vi "APOSGPS_String_To_Pos.vi"(8 "GPS IN":string="$GPGGA,080346.00,6343.152342,N,01104.396313,E,2,12,0.6,12.19,M,39.84,M,22.0,1007*4E", 11 "APOS IN":string="$PSIMSSB,170342.710,B34,A,,C,N,M,7.812,0.841,4.217,0.139,T,0.010904,") -> (2 "ROVpos":T1 caption="Real Matrix")   [LabVIEW 2012]
uses:
  <vilib>/Analysis/Matrix/Datatypes/RealMatrix.ctl
  <vilib>/imath/engines/lvmath2/RunTimeEngine/ErrorHandling/NIMS_Finalize Error.vi
  <vilib>/imath/engines/lvmath2/RunTimeEngine/Managers/WorkSpace/UID Generator.vi
  <vilib>/Analysis/Matrix/Numeric/Conversions/Matrix To Array - RM.vi
  <vilib>/imath/engines/lvmath2/RunTimeEngine/Managers/SymbolTable/Clear UID.vi
  <vilib>/imath/engines/lvmath2/RunTimeEngine/NodeEndStatement/NIMS_NodeEndStatement_Output.vi
  <instcachedir>/0/NIMS_NodeEndStatement_Output_53EC0D466D134D7ABD903AC30B43404B.lvgen/NIMS_NodeEndStatement_Output_53EC0D466D134D7ABD903AC30B43404B_012.vi
  <vilib>/Analysis/Matrix/Numeric/Conversions/Array To Matrix - RA2.vi
  <instcachedir>/0/NIMS_NodeEndStatement_Output_53EC0D466D134D7ABD903AC30B43404B.lvgen/NIMS_NodeEndStatement_Output_53EC0D466D134D7ABD903AC30B43404B_014.vi
  <vilib>/imath/engines/lvmath/Functions/Error Handling/MergeErrorsWrapper.vi
  <vilib>/imath/engines/lvmath2/RunTimeEngine/VariableToken/Read/NIMS_Get Elements - SorM(_,$) - Check.vi
  <instcachedir>/0/NIMS_Get Elements - SorM(_,$) - Check_FE352FA85B844FB785E5C28FDABD92A5.lvgen/NIMS_Get Elements - SorM(_,$) - Check_FE352FA85B844FB785E5C28FDABD92A5_000.vi
  <vilib>/imathl/engines/lvmath/Functions/Error Handling/Create Error.vi
  <vilib>/imath/engines/lvmath2/RunTimeEngine/RangeToken/NIMS_Range_R2.vi
  <vilib>/imath/engines/lvmath2/RunTimeEngine/ReplaceToken/NIMS_Replace - Check Row.vi
  <instcachedir>/0/NIMS_Replace - Check Row_8C35B66FE73A429EAC382AAA935851F0.lvgen/NIMS_Replace - Check Row_8C35B66FE73A429EAC382AAA935851F0_001.vi
  <vilib>/imath/engines/lvmath2/RunTimeEngine/ReplaceToken/NIMS_Replace - Size Check M(_,$)=VorM.vi
  <instcachedir>/0/NIMS_Replace - Size Check M(_,$)=VorM_05C8DDF28A13406EBCBD8C1ACDF4F548.lvgen/NIMS_Replace - Size Check M(_,$)=VorM_05C8DDF28A13406EBCBD8C1ACDF4F548_000.vi
  <vilib>/imath/engines/lvmath2/RunTimeEngine/ReplaceToken/NIMS_Replace - Assignment Check M(_,$)=VorM.vi
  <instcachedir>/0/NIMS_Replace - Assignment Check M(_,$)=VorM_DBF82BC42B054E2BA4F8E4D1989751AD.lvgen/NIMS_Replace - Assignment Check M(_,$)=VorM_DBF82BC42B054E2BA4F8E4D1989751AD_000.vi
  <vilib>/imath/engines/lvmath2/RunTimeEngine/VariableToken/Read/NIMS_Get Elements - RV(_) - Check.vi
  <instcachedir>/0/NIMS_Get Elements - RV(_) - Check_09E565EE58C54071A799578B82C9999A.lvgen/NIMS_Get Elements - RV(_) - Check_09E565EE58C54071A799578B82C9999A_000.vi
  <vilib>/imath/engines/lvmath2/RunTimeEngine/RunTimeType/NIMS_RunTimeType_From StrictType (excl LVString).vi
  <instcachedir>/0/NIMS_RunTimeType_From StrictType (excl LVString)_AC52D965D0864706932D20A05968E122.lvgen/NIMS_RunTimeType_From StrictType (excl LVString)_AC52D965D0864706932D20A05968E122_000.vi
  <vilib>/imath/engines/lvmath2/RunTimeEngine/ErrorHandling/NIMS_Create Error From Enums.vi
  <vilib>/imath/engines/lvmath2/RunTimeEngine/LocalVariableDefStatement/MC_LocalVariableDefStatement_Display.vi
  <vilib>/imath/engines/lvmath2/RunTimeEngine/RunTimeType/NIMS_RunTimeType_Set Source Original Bool.vi
  <vilib>/Analysis/Matrix/NI_Matrix.lvlib
  <vilib>/imath/engines/lvmath2/RunTimeEngine/Managers/SymbolTable/NIMS_WorkSpace.lvlib
panel:
  out "APOS String out":string
  out "GPS String out":string
  out "update":bool
  out "number of rows 2":i32
  out "number of rows":i32
  out "array 2":string[](array[string])
  out "array":string[](array[string])
  out "y":dbl
  out "x":dbl
  out "utmzone":string[](array[string])
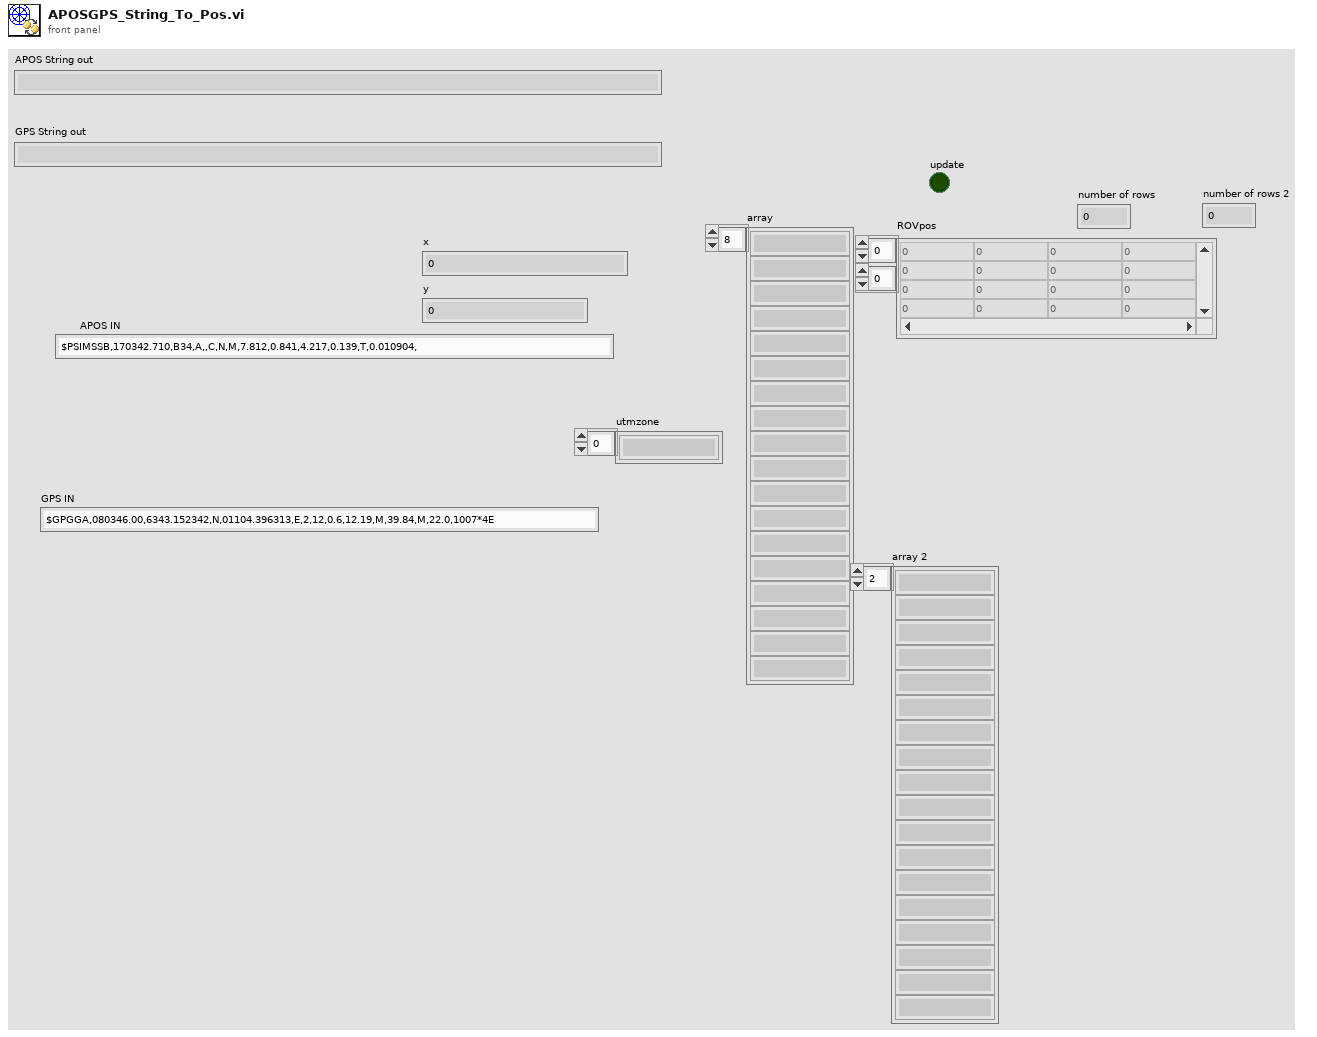
[diagram p1: front panel]
types:
  T1 = typedef "NI_Matrix.lvlib/RealMatrix.ctl" = dbl[][]
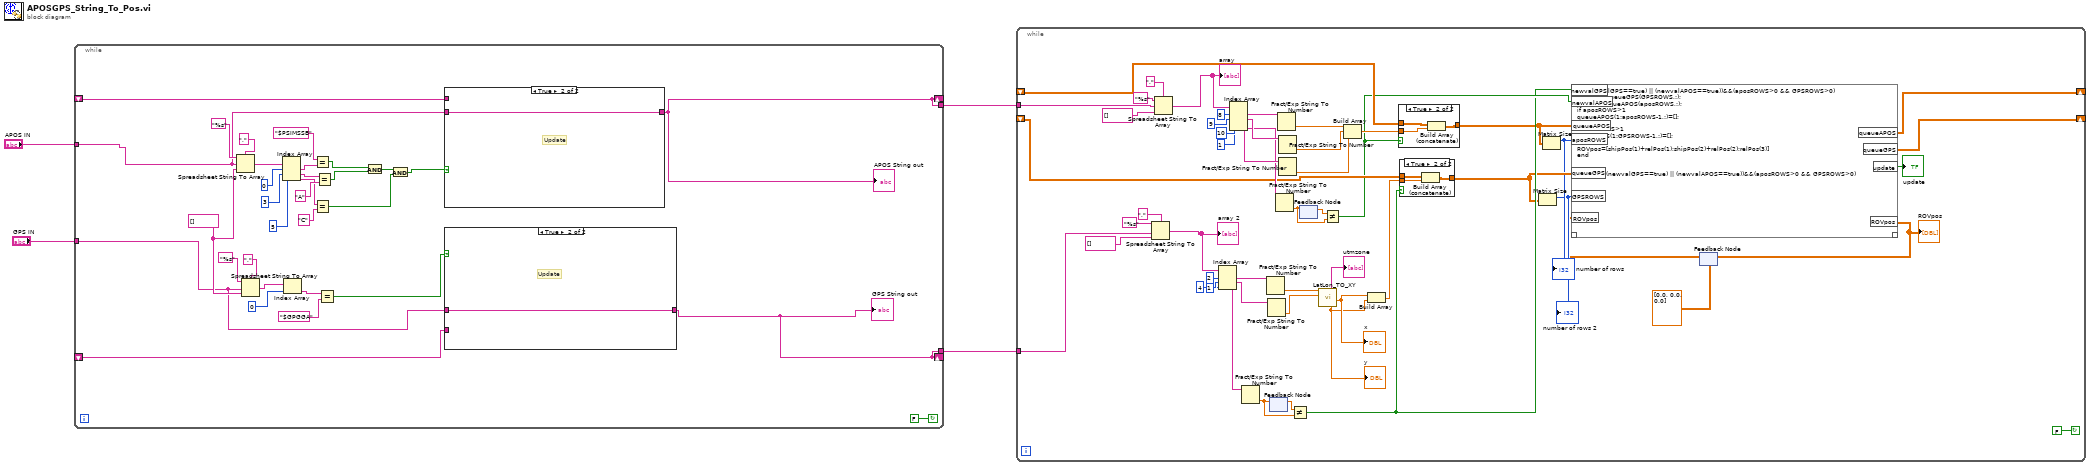
[diagram p0: block diagram]
diagram:
  n1 = while {
    shift-right: [w7] -> _
    shift-left: _ -> [w20]
    shift-right: [w8] -> _
    shift-left: _ -> [w16]
    tunnel: [w8] -> w4
    tunnel: [w7] -> w3
    tunnel: "APOS IN" -> [w6]
    tunnel: "GPS IN" -> [w5]
    stop <- FALSE continue-if-true
    w33 = string[] []
    n2 = Spreadsheet String To Array(delimiter (Tab)=",", format string="%s", spreadsheet string=w6, array type (2D Dbl)=w33) -> (array=w31:string[])
    n3 = Spreadsheet String To Array(delimiter (Tab)=",", format string="%s", spreadsheet string=w5, array type (2D Dbl)=w33) -> (array=w34:string[])
    n4 = Index Array(array=w31, index #1=0, index #2=3, index #3=5) -> (element #1=w25:string, element #2=w23:string, element #3=w13:string)
    n5 = Index Array(array=w34, index=0) -> (element=w19:string)
    n6 = Equal?(x="$PSIMSSB", y=w25) -> (x = y?=w22:bool)
    n7 = Equal?(x=w13, y="C") -> (x = y?=w10:bool)
    n8 = Equal?(x=w23, y="A") -> (x = y?=w21:bool)
    n9 = Equal?(x=w19, y="$GPGGA") -> (x = y?=w17:bool)
    n10 = And(x=w22, y=w21) -> (x .and. y?=w11:bool)
    n11 = And(x=w11, y=w10) -> (x .and. y?=w9:bool)
    n12 = case shown="True" w9 {
      tunnel: w6 -> [_ w40]
      tunnel: [w39 w40] -> w7
      tunnel: w20 -> [w39 _]
      frame False {
        # "Keep old value"
      }
      frame True {
        # "Update"
      }
    }
    "APOS String out" <- w7
    n13 = case shown="True" w17 {
      tunnel: w5 -> [_ w38]
      tunnel: [w37 w38] -> w8
      tunnel: w16 -> [w37 _]
      frame False {
        # "keep old value"
      }
      frame True {
        # "Update"
      }
    }
    "GPS String out" <- w8
  }
  n14 = while {
    shift-right: [w47] -> _
    shift-left: _ -> [w56]
    shift-right: [w46] -> _
    shift-left: _ -> [w58]
    tunnel: w4 -> [w43]
    tunnel: w3 -> [w42]
    stop <- FALSE continue-if-true
    n15 = Spreadsheet String To Array(delimiter (Tab)=",", format string="%s", spreadsheet string=w43, array type (2D Dbl)=string[] [] ("Array")) -> (array=w78:string[])
    "array 2" <- w78
    n16 = Spreadsheet String To Array(delimiter (Tab)=",", format string="%s", spreadsheet string=w42, array type (2D Dbl)=string[] [] ("Array")) -> (array=w89:string[])
    "array" <- w89
    n17 = Index Array(array=w78, index #1=2 ("index"), index #2=4 ("index"), index #3=1 ("index")) -> (element #1=w81:string, element #2=w82:string, element #3=w65:string)
    n18 = Index Array(array=w89, index #1=8 ("index"), index #2=9 ("index"), index #3=10 ("index"), index #4=1 ("index")) -> (element #1=w85:string, element #2=w84:string, element #3=w83:string, element #4=w64:string)
    n19 = Fract/Exp String To Number(string=w65) -> (number=w60:dbl)  [unwired: 3 in, 1 out]
    n20 = Fract/Exp String To Number(string=w81) -> (number=w74:dbl)  [unwired: 3 in, 1 out]
    n21 = Fract/Exp String To Number(string=w82) -> (number=w73:dbl)  [unwired: 3 in, 1 out]
    n22 = feedback-in #1(w60) -> ()
    n23 = feedback #1() -> (w63:dbl)  [unwired: 1 in]
    n24 = Fract/Exp String To Number(string=w64) -> (number=w61:dbl)  [unwired: 3 in, 1 out]
    n25 = Fract/Exp String To Number(string=w85) -> (number=w70:dbl)  [unwired: 3 in, 1 out]
    n26 = Fract/Exp String To Number(string=w84) -> (number=w69:dbl)  [unwired: 3 in, 1 out]
    n27 = Fract/Exp String To Number(string=w83) -> (number=w68:dbl)  [unwired: 3 in, 1 out]
    n28 = Not Equal?(x=w63, y=w60) -> (x != y?=w54:bool)
    n29 = feedback #2() -> (w62:dbl)  [unwired: 1 in]
    n30 = feedback-in #2(w61) -> ()
    n31 = call "LatLon_TO_XY.vi"("Longitude"=w73, "Latitude"=w74) -> ("x"=w72:dbl, "y"=w71:dbl, "utmzone"=→"utmzone":string[])  [unwired: 7 in]
    "x" <- w72
    "y" <- w71
    n32 = Not Equal?(x=w62, y=w61) -> (x != y?=w55:bool)
    n33 = Build Array(w70, w69, w68) -> (w59:dbl[])
    n34 = Build Array(w72, w71) -> (w57:dbl[])
    n35 = case shown="True" w55 {
      tunnel: w59 -> [_ w100]
      tunnel: w58 -> [w98 w101]
      tunnel: [w98 w99] -> w53
      frame False {
      }
      frame True {
        n36 = Build Array (concatenate)(w101, w100) -> (w99:T1)
      }
    }
    n37 = case shown="True" w54 {
      tunnel: w57 -> [_ w96]
      tunnel: w56 -> [w94 w95]
      tunnel: [w94 w97] -> w52
      frame False {
      }
      frame True {
        n38 = Build Array (concatenate)(w95, w96) -> (w97:T1)
      }
    }
    n39 = Matrix Size(0:w52) -> (1:w50:i32)  [unwired: 1 out]
    "number of rows 2" <- w50
    n40 = Matrix Size(0:w53) -> (1:w51:i32)  [unwired: 1 out]
    "number of rows" <- w51
    n41 = feedback #3(T1 [[0.0], [0.0], [0.0]] ("ROVpos")) -> (w48:T1)
    n42 = mathscript code="if ((newvalGPS==true) || (newvalAPOS==true))&&(aposROWS>0 && GPSROWS>0)\nshipPos=queueGPS(GPSROWS,:);\nrelPos=queueAPOS(aposROWS,:);\nif aposROWS>1\nqueueAPOS(1:aposROWS-1,:)=[];\nend\nif GPSROWS>1\nqueueGPS(1:GPSROWS-1,:)=[];\nend\nROVpos=[shipPos(1)+relPos(1);shipPos(2)+relPos(2);relPos(3)]\nend \n\n\nupdate=((newvalGPS==true) || (newvalAPOS==true))&&(aposROWS>0 && GPSROWS>0)"("newvalGPS"=w54, "newvalAPOS"=w55, "queueAPOS"=w53, "queueGPS"=w52, "aposROWS"=w51, "GPSROWS"=w50, "ROVpos"=w48) -> ("ROVpos"=w49:T1, "queueAPOS"=w46:T1, "queueGPS"=w47:T1, "update"=→"update":bool)  [unwired: 1 in, 1 out]
    "ROVpos" <- w49
    n43 = feedback-in #3(w49) -> ()
  }
